vi "AD5627R_Ref.vi"(2 "error in (no error)":errorcluster, 5 "RIO Device":T1) -> (0 "error out":errorcluster, 1 "RIO Device out":T1)   [LabVIEW 2018]
uses:
  <vilib>/userdefined/High Color/nirio_resource_hc.ctl
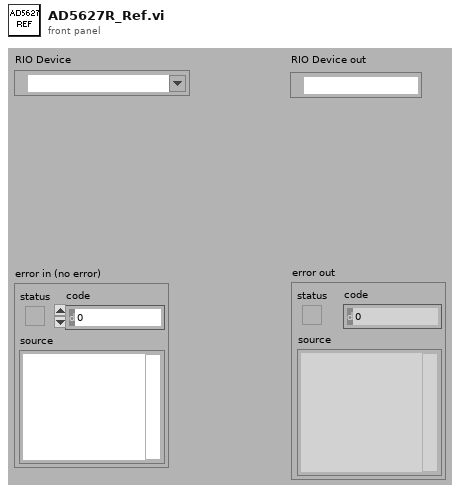
[diagram p1: front panel]
types:
  T1 = typedef "nirio_resource_hc.ctl" = tag
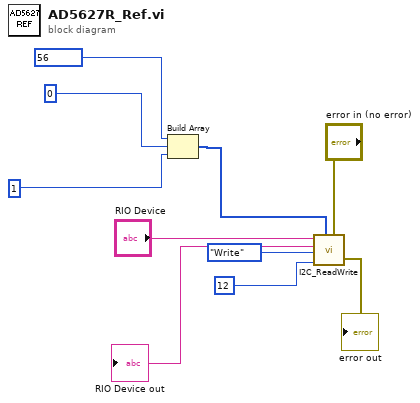
[diagram p0: block diagram]
diagram:
  n1 = Build Array(u8 56 ("x"), u8 0 ("x"), u8 1 ("x")) -> (w6:u8[])
  n2 = call "I2C_ReadWrite.vi"("error in (no error)"="error in (no error)", "DataWriteArray"=w6, "Address"=u8 12, "Command"=enum16{"Write", "Read"}."Write", "RIO Device"="RIO Device") -> ("error out"=→"error out":errorcluster, "RIO Device out"=→"RIO Device out":T1)  [unwired: 4 in, 1 out]
